vi "Example (subVI).vi"() -> ()   [LabVIEW 2021]
panel:
  in  "stop":bool
  out "°C":dbl(slide) scale=0.0..100.0
  in  "°F":dbl(slide) scale=0.0..250.0
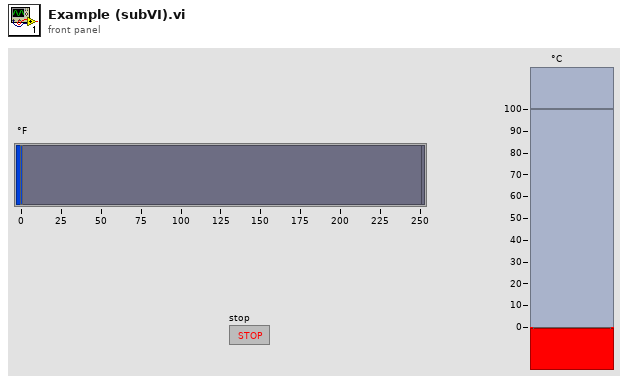
[diagram p1: front panel]
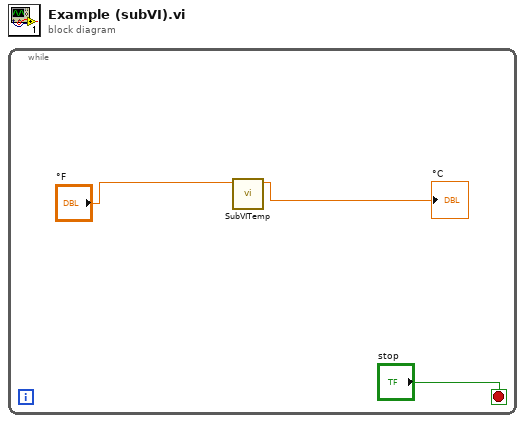
[diagram p0: block diagram]
diagram:
  n1 = while {
    stop <- "stop" stop-if-true
    n2 = call "SubVITemp.vi"("°F"="°F") -> ("Numeric"=→"°C":dbl)  [unwired: 10 in]
  }
